vi "Utility Head ID.vi"(5 "Retry Attempts (0)":i32 min=0, 7 "Fast Comms (F)":bool, 8 "error in (no error)":errorcluster, 11 "VISA resource name":refnum<visa-resource-name>) -> (0 "error out":errorcluster, 2 "Head ID":string, 3 "VISA resource name out":refnum<visa-resource-name>)   [LabVIEW 2020, in "driver_chromtech_next_gen.lvlib"]
doc: "Query the pump for the current Head ID."
uses:
  driver_chromtech_next_gen.lvlib
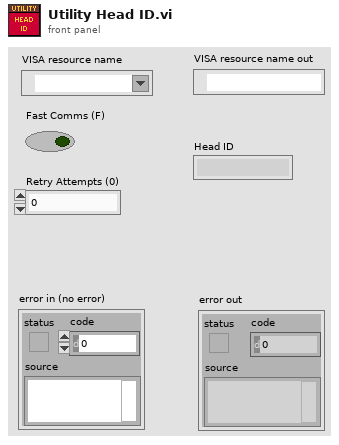
[diagram p1: front panel]
types:
  T1 = cluster{"Flow rate":dbl, "Running":bool, "Pressure Comp":i32, "Head ID":string, "Upper Pressure Fault":bool, "Lower Pressure Fault":bool, "In Prime":bool, "Keypad Enabled":bool, "Motor Stall Fault":bool}
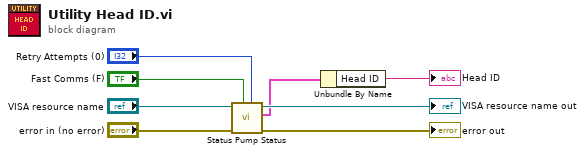
[diagram p0: block diagram]
diagram:
  n1 = call "Status Pump Status.vi"("Retry Attempts (0)"="Retry Attempts (0)", "Fast Comms (F)"="Fast Comms (F)", "error in (no error)"="error in (no error)", "VISA resource name"="VISA resource name") -> ("error out"=→"error out":errorcluster, "Status Cluster"=w3:T1, "VISA resource name out"=→"VISA resource name out":refnum<visa-resource-name>)  [unwired: 5 in]
  n2 = Unbundle By Name(w3) -> ("Head ID"=→"Head ID":string)
